vi "get_gpu_info.vi"(8 "Error in":errorcluster caption="Error in (no error)") -> (0 "Error out":errorcluster, 3 "GPU Info":string)   [LabVIEW 2018]
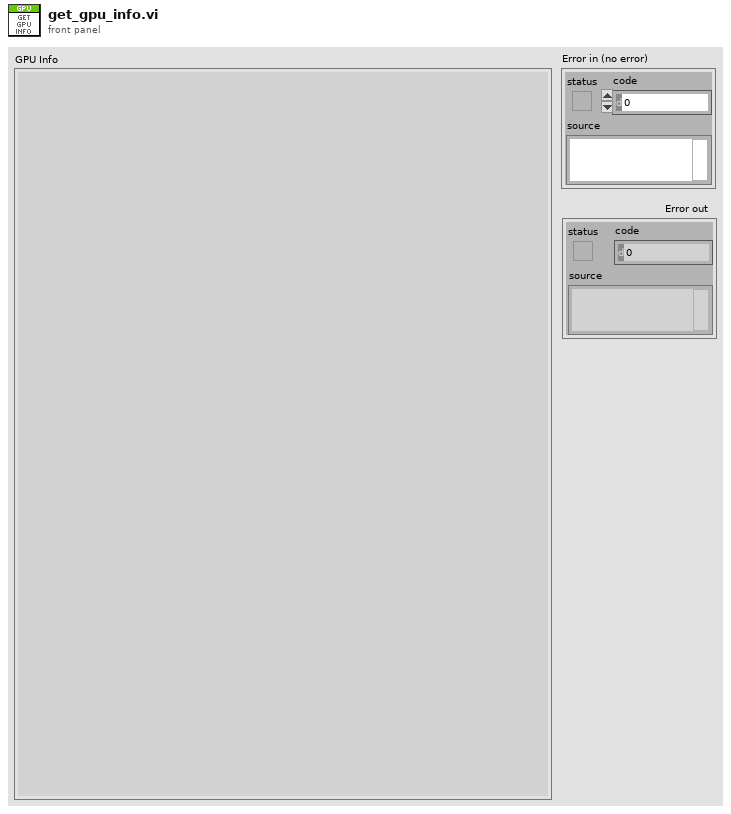
[diagram p1: front panel]
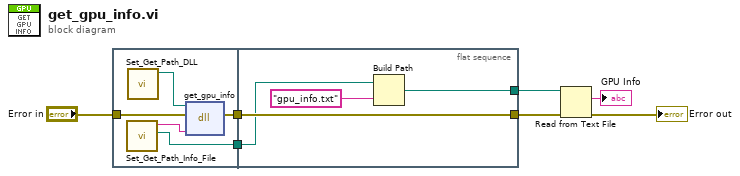
[diagram p0: block diagram]
diagram:
  n1 = flat-sequence {
    tunnel: "Error in" -> [w12]
    tunnel: [w11] -> w3
    tunnel: [w8] -> w1
    tunnel: [w16] -> w5
    tunnel: w3 -> [w16]
    tunnel: [w14] -> w2
    tunnel: w1 -> [w13]
    frame #0 {
      n2 = call "Set_Get_Path_Info_File.vi"() -> ("Info File Path Out"=w8:path, "Info Path File Out"=w9:string)  [unwired: 10 in]
      n3 = call "Set_Get_Path_DLL.vi"() -> ("path DLL Out"=w10:path)  [unwired: 11 in]
      n4 = dll-call lib="C:/Users/AUTIS/Documents/TFG/Proyecto/Visual Studio/SR_GPU_TOOLKIT_INIT/x64/Release/SR_GPU_TOOLKIT.dll" fn="get_gpu_info"(path in=w10, error in=w12, "url"=w9) -> (error out=w11:errorcluster)  [unwired: 3 in, 1 out]
    }
    frame #1 {
      n5 = Build Path(base path=w13, name or relative path="gpu_info.txt") -> (appended path=w14:path)
    }
  }
  n6 = Read from Text File(file (use dialog)=w2, error in=w5) -> (text=→"GPU Info":string, error out=→"Error out":errorcluster)  [unwired: 2 in, 2 out]
